vi "Write Waveform Array.vi"(8 "error in (no error)":errorcluster, 10 "Waveform Array":waveform(dbl)[](array[waveform]), 11 "Waveform Array Result in":refnum<class "Waveform Array Result.lvclass">) -> (0 "error out":errorcluster, 3 "Waveform Array Result out":refnum<class "Waveform Array Result.lvclass">)   [LabVIEW 2015, in "Waveform Array Result.lvclass"]
uses:
  Waveform Array Result.lvclass
  Waveform Array Result.lvclass/Waveform Array Result.ctl
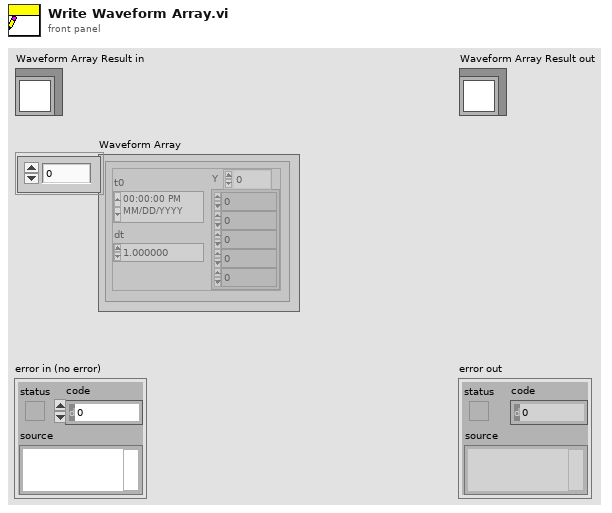
[diagram p1: front panel]
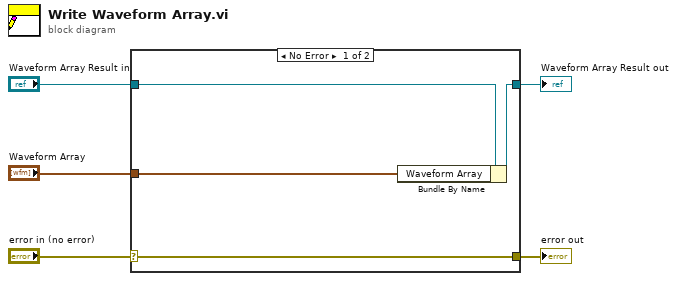
[diagram p0: block diagram]
diagram:
  n1 = case shown="No Error" "error in (no error)" {
    selector: "error in (no error)" -> [w9 w10]
    tunnel: [w9 w10] -> w4
    tunnel: [w7 w11] -> w2
    tunnel: "Waveform Array Result in" -> [w8 w11]
    tunnel: "Waveform Array" -> [w6 _]
    frame No Error {
      n2 = Bundle By Name(cluster=w8, "Waveform Array"=w6) -> (w7:refnum<class "Waveform Array Result.lvclass">)
    }
    frame Error {
    }
  }
  "error out" <- w4
  "Waveform Array Result out" <- w2
